vi "ARydh_set_frequency -- V1.vi"(4 "Oscillator (0)":u16, 8 "Error In":errorcluster, 9 "timeconstant (s)":dbl=0.006, 10 "Freq in (Hz)":dbl=40000.0 format="%#_13g", 11 "MCL object":T1) -> (0 "Error Out":errorcluster, 1 "z out (V)":cdb, 2 "Freq out (Hz)":dbl=40000.0 format="%#_13g", 3 "MCL object OUT":T1)   [LabVIEW 2018]
uses:
  Users/Nanocal/Desktop/Calorimetry v1.3/MCL.lvlibp/MCL library/MCL_DataRef.ctl
  Users/Nanocal/Desktop/Calorimetry v1.3/MCL.lvlibp/SynkTek FPGA/FPGA_SharedResources/FPGASharedResources_FreqCtrl_FreqGenTypedef.ctl
  Users/Nanocal/Desktop/Calorimetry v1.3/MCL.lvlibp
  Users/Nanocal/Desktop/Calorimetry v1.3/MCL.lvlibp/SynkTek FPGA/FPGA_SharedResources/FPGA_SharedResources.lvlib
  Users/Nanocal/Desktop/Calorimetry v1.3/MCL.lvlibp/SynkTek Host/LIControl/LIControl_LockinTimeConstant_typedef.ctl
  Users/Nanocal/Desktop/Calorimetry v1.3/MCL.lvlibp/SynkTek Host/LIControl/LIControl.lvlib
  Users/Nanocal/Desktop/Calorimetry v1.3/MCL.lvlibp/SynkTek Host/LIControl/LIControl_FreqCtrl_typedef.ctl
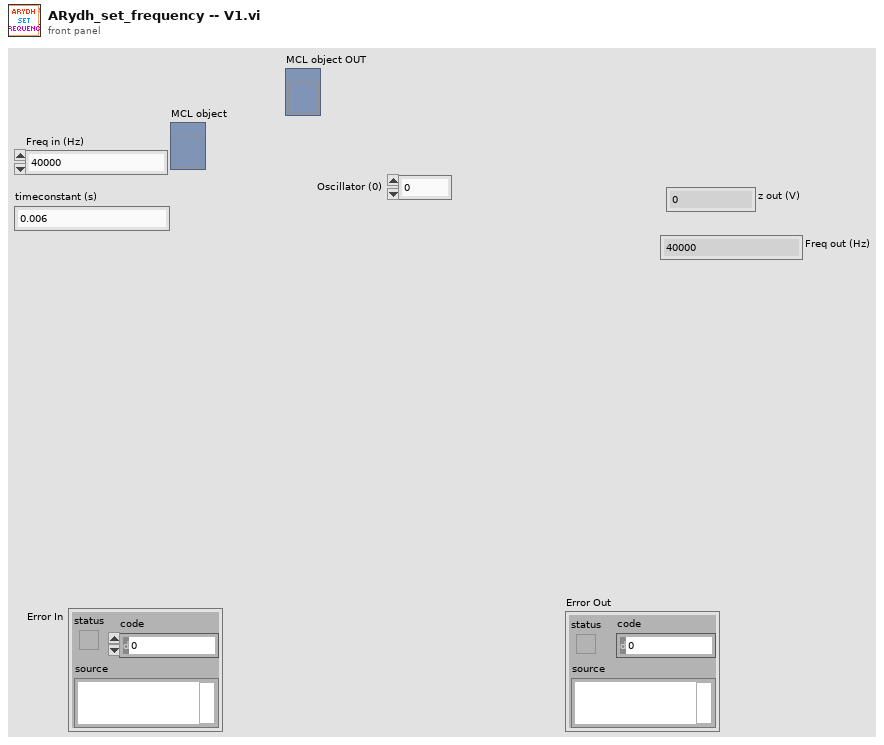
[diagram p1: front panel]
types:
  T1 = typedef "MCL.lvlibp/MCL_DataRef.ctl" = refnum<vi>
  T2 = typedef "MCL.lvlibp/FPGA_SharedResources.lvlib/FPGASharedResources_FreqCtrl_FreqGenTypedef.ctl" = enum8{"Frequency 1", "Frequency 2", "Frequency 3", "Frequency 4", "Frequency 5", "Frequency 6: PLL 1", "Frequency 7: PLL 2", "Frequency 8"}
  T3 = typedef "MCL.lvlibp/LIControl.lvlib/LIControl_FreqCtrl_typedef.ctl" = cluster{"Frequency (Hz)":dbl, "Ramp changes":bool, "Ramp time const. (s)":T4}
  T4 = typedef "MCL.lvlibp/LIControl.lvlib/LIControl_LockinTimeConstant_typedef.ctl" = dbl
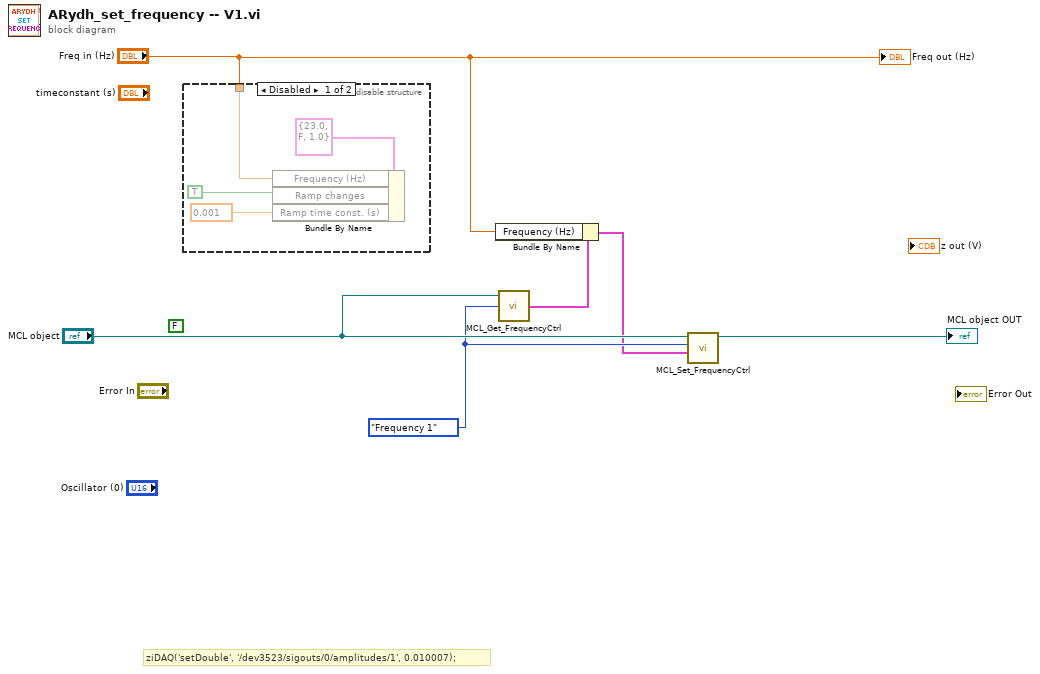
[diagram p0: block diagram]
diagram:
  w4 = FPGASharedResources_FreqCtrl_FreqGenTypedef."Frequency 1" ("Frequency generator")
  (unwired) FALSE
  # "ziDAQ('setDouble', '/dev3523/sigouts/0/amplitudes/1', 0.010007);"
  n1 = disable-structure shown="Disabled" {
    disable-tunnel: "Freq in (Hz)" -> [w7 _]
    frame Disabled {
      w8 = T4 0.001 items=["100 s"=100.0, "50 s"=50.0, "20 s"=20.0, "10 s"=10.0, "5 s"=5.0, "3 s"=3.0, "2 s"=2.0, "1 s"=1.0, "0.5 s"=0.5, "0.3 s"=0.3, "0.2 s"=0.2, "0.1 s"=0.1, "50 ms"=0.05, "20 ms"=0.02, "10 ms"=0.01, "5 ms"=0.005, "2 ms"=0.002, "1 ms"=0.001] ("Ramp time const. (s)")
      n2 = Bundle By Name(cluster=T3 {"Frequency (Hz)"=23.0, "Ramp changes"=FALSE, "Ramp time const. (s)"=1.0} ("FrequencyCtrl"), "Frequency (Hz)"=w7, "Ramp changes"=TRUE, "Ramp time const. (s)"=w8) -> ()  [unwired: 1 out]
    }
    frame Enabled {
    }
  }
  n3 = call "MCL_Get_FrequencyCtrl.vi"("Frequency generator"=w4, "MCL object"="MCL object") -> ("FrequencyCtrl"=w3:T3)  [unwired: 1 in, 2 out]
  n4 = Bundle By Name(cluster=w3, "Frequency (Hz)"="Freq in (Hz)") -> (w2:T3)
  n5 = call "MCL_Set_FrequencyCtrl.vi"("FrequencyCtrl"=w2, "Frequency generator"=w4, "MCL object"="MCL object") -> ("MCL object"=→"MCL object OUT":T1)  [unwired: 3 in, 1 out]
  "Freq out (Hz)" <- "Freq in (Hz)"
